vi "Test Multiple IDs Server.vi"() -> ()   [LabVIEW 2020]
uses:
  TCP Comms/State.ctl
  Slider ID.ctl
  0ccc8330-39ba-48a1-8223-cf5070bef32b.vi
  56c8a86d-a319-4de7-adfb-b6a856ff4293.vi
  259ed48f-7e9e-4079-aa69-b33d26c51f3a.vi
  <vilib>/Utility/error.llb/Clear Errors.vi
  TCP Comms/Get Connected.vi
  <vilib>/Utility/error.llb/Error Cluster From Error Code.vi
  TCP Comms/Connection Ref.vi
  TCP Comms/Close TCP.vi
  TCP Comms/TCP Comms.lvlib
panel:
  out "Read Period":dbl
  in  "Close":bool
  in  "Open":bool
  out "Server Error":errorcluster
  out "Server State":T1
  out "Slider B (Client)":dbl(slide) scale=0.0..10.0
  out "Slider A (Client)":i32(slide) scale=0.0..10.0
  in  "Slider D (Server)":i8(slide) scale=0.0..10.0
  in  "Slider C (Server)":u16(slide) scale=0.0..10.0
  # "Run this VI and then click Open Server to open the connection for the client to connect. Connections can be open in any order and once the connection is established, the values will start being sent to and read from the connected client.\n\nClose Server closes the connection but leaves the app running and the server can be opened again."
  # "Close the window to stop the server"
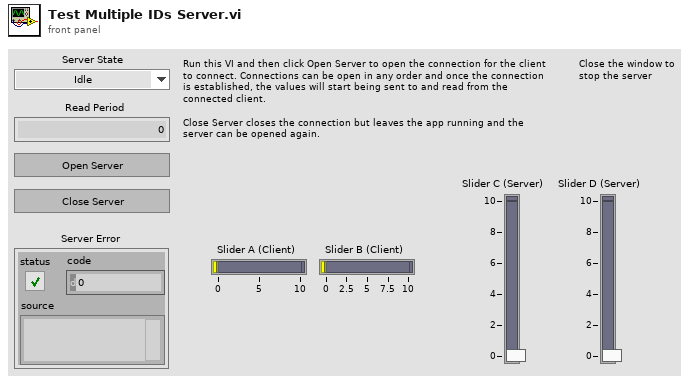
[diagram p1: front panel]
types:
  T1 = typedef "TCP Comms.lvlib/State.ctl" = enum16{"Idle", "Starting", "Connecting", "Connected", "Disconnecting", "Stopped"}
  T2 = typedef "TCP Comms.lvlib/TCP Comm.ctl" = refnum<data-value>
  T3 = typedef "Slider ID.ctl" = enum16{"Slider A", "Slider B", "Slider C", "Slider D"}
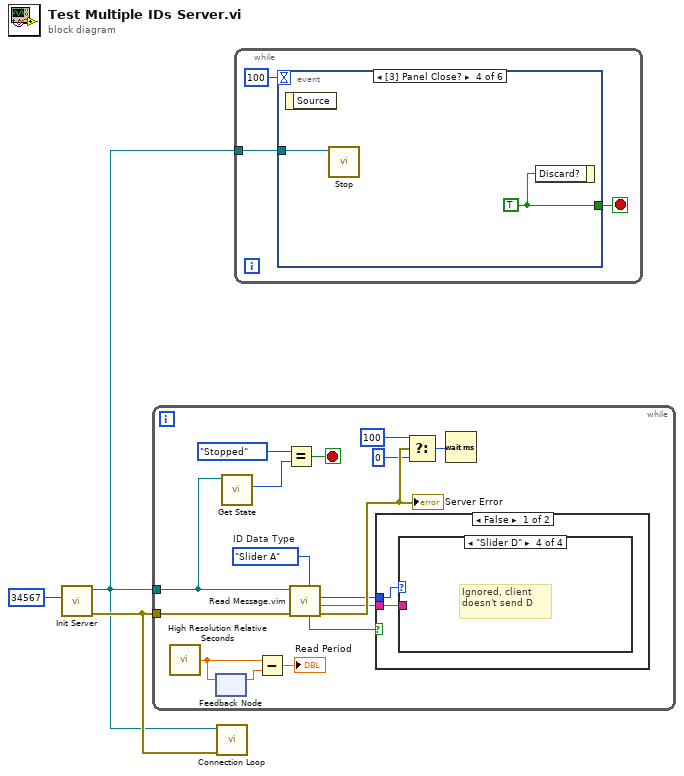
[diagram p0: block diagram]
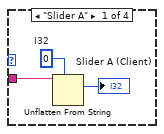
[diagram p2: hidden frame]
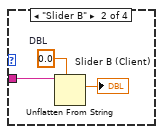
[diagram p3: hidden frame]
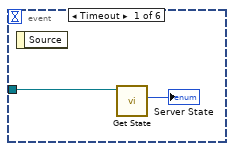
[diagram p6: hidden frame]
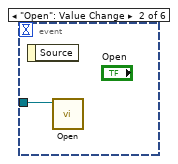
[diagram p7: hidden frame]
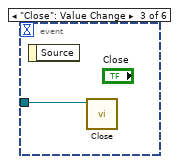
[diagram p8: hidden frame]
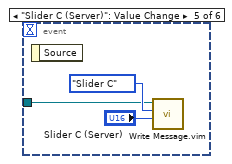
[diagram p9: hidden frame]
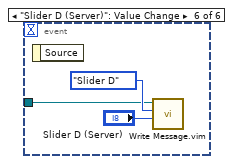
[diagram p10: hidden frame]
diagram:
  n1 = call "Init Server.vi"("Port"=u16 34567) -> ("error out"=w3:errorcluster, "TCP Comm"=w1:T2)  [unwired: 9 in]
  n2 = while {
    tunnel: w1 -> [w5]
    tunnel: w3 -> [w4]
    stop <- w16 stop-if-true
    w15 = Slider_ID."Slider A"  # ID Data Type
    n3 = call <vilib>:"High Resolution Relative Seconds.vi"() -> ("relative seconds"=w11:dbl)
    n4 = feedback-in #1(w11) -> ()
    n5 = feedback #1() -> (w10:dbl)  [unwired: 1 in]
    n6 = call "Get State.vi"("TCP Comm In"=w5) -> ("State"=w18:T1)  [unwired: 9 in, 1 out]
    n7 = Subtract(x=w11, y=w10) -> (x-y=→"Read Period":dbl)
    n8 = Equal?(x=State."Stopped", y=w18) -> (x = y?=w16:bool)
    n9 = call "Read Message.vim"("Message ID Data Type (String)"=w15, "error in (no error)"=w4, "TCP Comm In"=w5) -> ("error out"=w19:errorcluster, "Data"=w12:string, "Message ID"=w13:T3, "Timeout?"=w14:bool)  [unwired: 3 in, 2 out]
    "Server Error" <- w19
    n10 = case shown="False" w14 {
      tunnel: w13 -> [w21 _]
      tunnel: w12 -> [w20 _]
      frame False {
        n11 = case shown="\"Slider D\"" w21 {
          tunnel: w20 -> [w23 w26 _ _]
          frame "Slider A" {
            w24 = 0  # I32
            n12 = Unflatten From String(type=w24, binary string=w23) -> (value=→"Slider A (Client)":i32)  [unwired: 3 in, 2 out]
          }
          frame "Slider B" {
            w27 = 0.0  # DBL
            n13 = Unflatten From String(type=w27, binary string=w26) -> (value=→"Slider B (Client)":dbl)  [unwired: 3 in, 2 out]
          }
          frame "Slider C" {
            # "Ignored, client doesn't send C"
          }
          frame "Slider D" {
            # "Ignored, client doesn't send D"
          }
        }
      }
      frame True {
      }
    }
    n14 = Select(t=u32 100, s=w19, f=u32 0 ("milliseconds to wait")) -> (s? t:f=w7:u32)
    n15 = Wait (ms)(milliseconds to wait=w7) -> ()  [unwired: 1 out]
  }
  n16 = call "Connection Loop.vi"("error in (no error)"=w3, "TCP Comm"=w1) -> ()  [unwired: 9 in, 1 out]
  n17 = while {
    tunnel: w1 -> [w30]
    stop <- w29 stop-if-true
    n18 = event shown="[3] Panel Close?" {
      selector: _ -> [_ _ _ _ _ _]
      dyn-events: _ -> [_ _ _ _ _ _]
      timeout: 100 -> [_ _ _ _ _ _]
      tunnel: w30 -> [w32 w33 w34 w36 w38 w41]
      tunnel: [_ _ _ w35 _ _] -> w29
      event Timeout {
        n19 = event-data() -> ()  [unwired: 1 in, 1 out]
        n20 = call "Get State.vi"("TCP Comm In"=w32) -> ("State"=→"Server State":T1)  [unwired: 9 in, 1 out]
      }
      event "Open": Value Change {
        n21 = event-data() -> ()  [unwired: 1 in, 1 out]
        n22 = call "Open.vi"("TCP Comm"=w33) -> ()  [unwired: 10 in, 1 out]
      }
      event "Close": Value Change {
        n23 = event-data() -> ()  [unwired: 1 in, 1 out]
        n24 = call "Close.vi"("TCP Comm"=w34) -> ()  [unwired: 10 in, 1 out]
      }
      event Panel Close? {
        w35 = TRUE
        n25 = event-data() -> ()  [unwired: 1 in, 1 out]
        n26 = call "Stop.vi"("TCP Comm"=w36) -> ()  [unwired: 10 in, 1 out]
        n27 = event-data("Discard?"=w35) -> ()  [unwired: 1 in, 1 out]
      }
      event "Slider C (Server)": Value Change {
        n28 = event-data() -> ()  [unwired: 1 in, 1 out]
        n29 = call "Write Message.vim"("Data"="Slider C (Server)", "Message ID (None)"=Slider_ID."Slider C" ("Slider ID"), "TCP Comm In"=w38) -> ()  [unwired: 6 in, 3 out]
      }
      event "Slider D (Server)": Value Change {
        n30 = event-data() -> ()  [unwired: 1 in, 1 out]
        n31 = call "Write Message.vim"("Data"="Slider D (Server)", "Message ID (None)"=Slider_ID."Slider D" ("Slider ID"), "TCP Comm In"=w41) -> ()  [unwired: 6 in, 3 out]
      }
    }
  }
